vi "Revision Query.vi"(0 "VISA resource name":refnum<visa-resource-name>, 11 "error in (no error)":errorcluster) -> (4 "VISA resource name out":refnum<visa-resource-name>, 6 "Instrument Driver Revision":string, 8 "Instrument Hardware Revision":dbl, 10 "Instrument Firmware Revision":dbl, 15 "error out":errorcluster)   [LabVIEW 2020, in "MagnaDC.lvlib"]
doc: "Queries the current instrument firmware revision and instrument driver revision.\n\nRefer to the Readme file for detailed driver information including modification history."
uses:
  MagnaDC.lvlib
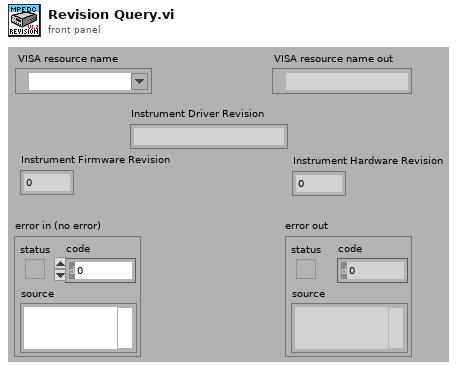
[diagram p1: front panel]
types:
  T1 = enum32{"invalid app kind", "Development System", "Run Time System", "Student Edition", "Embedded LabVIEW", "Evaluation", "Custom"}
  T2 = cluster{"Major":u16, "Minor":u16, "Fix":u16, "Build":u16}
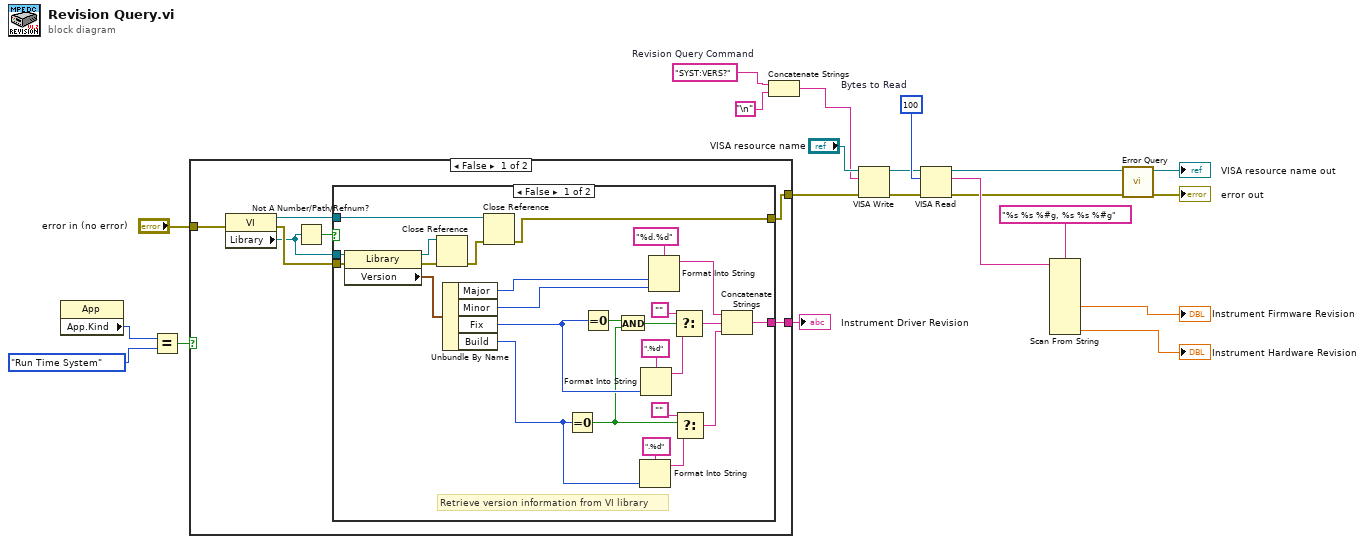
[diagram p0: block diagram]
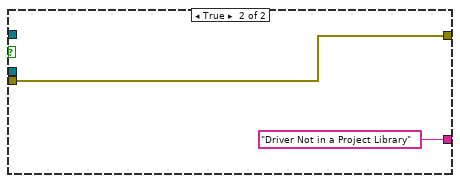
[diagram p2: hidden frame]
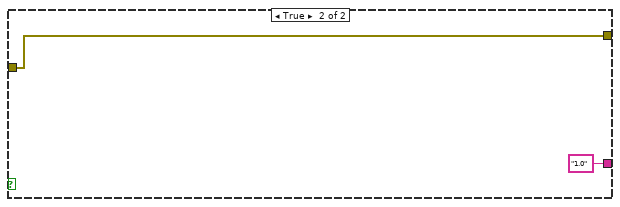
[diagram p3: hidden frame]
diagram:
  w3 = "SYST:VERS?"  # Revision Query Command
  w20 = u32 100  # Bytes to Read
  n1 = property class="App"() -> ("App.Kind"=w7:T1)  [unwired: 2 in, 2 out]
  n2 = Equal?(x=w7, y=T1."Run Time System" ("Application:Kind")) -> (x = y?=w8:bool)
  n3 = case shown="False" w8 {
    tunnel: [w24 "1.0"] -> w11
    tunnel: "error in (no error)" -> [w23 w57]
    tunnel: [w22 w57] -> w9
    frame False {
      n4 = property class="VI"(error in=w23) -> (reference out=w28:refnum<vi>, error out=w27:errorcluster, "Library"=w26:refnum<vi>)  [unwired: 1 in]
      n5 = Not A Number/Path/Refnum?(number/path/refnum=w26) -> (NaN/Path/Refnum?=w25:bool)
      n6 = case shown="False" w25 {
        tunnel: w28 -> [w51 _]
        tunnel: w27 -> [w36 w56]
        tunnel: [w31 w56] -> w22
        tunnel: [w30 "Driver Not in a Project Library"] -> w24
        tunnel: w26 -> [w29 _]
        frame False {
          # "Retrieve version information from VI library"
          n7 = property class="Library"(reference=w29, error in=w36) -> (reference out=w53:refnum<vi>, error out=w54:errorcluster, "Version"=w50:T2)
          n8 = Close Reference(reference=w53, error in (no error)=w54) -> (error out=w52:errorcluster)
          n9 = Unbundle By Name(w50) -> ("Major"=w39:u16, "Minor"=w38:u16, "Fix"=w35:u16, "Build"=w37:u16)
          n10 = Close Reference(reference=w51, error in (no error)=w52) -> (error out=w31:errorcluster)
          n11 = Equal To 0?(x=w37) -> (x = 0?=w33:bool)
          n12 = Equal To 0?(x=w35) -> (x = 0?=w34:bool)
          n13 = And(x=w34, y=w33) -> (x .and. y?=w32:bool)
          n14 = Format Into String(format string=".%d", w37) -> (resulting string=w43:string)  [unwired: 2 in, 1 out]
          n15 = Format Into String(format string=".%d", w35) -> (resulting string=w47:string)  [unwired: 2 in, 1 out]
          n16 = Format Into String(format string="%d.%d", w39, w38) -> (resulting string=w45:string)  [unwired: 2 in, 1 out]
          n17 = Select(t="", s=w32, f=w47) -> (s? t:f=w44:string)
          n18 = Select(t="", s=w33, f=w43) -> (s? t:f=w40:string)
          n19 = Concatenate Strings(w45, w44, w40) -> (w30:string)
        }
        frame True {
        }
      }
    }
    frame True {
    }
  }
  "Instrument Driver Revision" <- w11
  n20 = Concatenate Strings(w3, "\n") -> (w1:string)
  n21 = VISA Write(VISA resource name="VISA resource name", write buffer=w1, error in (no error)=w9) -> (VISA resource name out=w19:refnum<visa-resource-name>, error out=w18:errorcluster)  [unwired: 1 out]
  n22 = VISA Read(VISA resource name=w19, byte count=w20, error in (no error)=w18) -> (VISA resource name out=w14:refnum<visa-resource-name>, read buffer=w17:string, error out=w15:errorcluster)  [unwired: 1 out]
  n23 = Scan From String(format string="%s %s %#g, %s %s %#g", input string=w17) -> (output 3=→"Instrument Firmware Revision":dbl, output 6=→"Instrument Hardware Revision":dbl)  [unwired: 12 in, 3 out]
  n24 = call "Error Query.vi"("error in (no error)"=w15, "VISA resource name"=w14) -> ("error out"=→"error out":errorcluster, "VISA resource name out"=→"VISA resource name out":refnum<visa-resource-name>)  [unwired: 6 in, 2 out]
